vi "Value_Update_to_Preset.vi"(9 "Coordinate Array with Changes":i32[][](array[numeric]), 11 "Input Table":string[][](array[string])) -> (1 "Column Headers":string[](array[string])=["Device Name", "Device Variable", "Preset Value"], 3 "Output Table with Changes":string[][](array[string]))   [LabVIEW 2020]
uses:
  <userlib>/_OpenG.lib/array/array.llb/Empty 2D Array (I32)__ogtk.vi
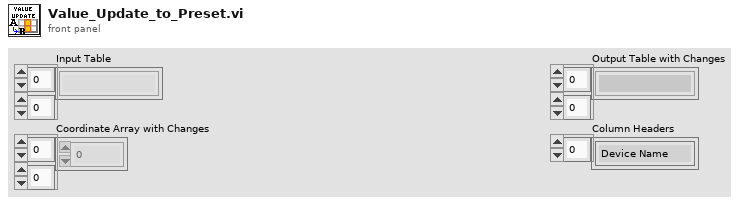
[diagram p1: front panel]
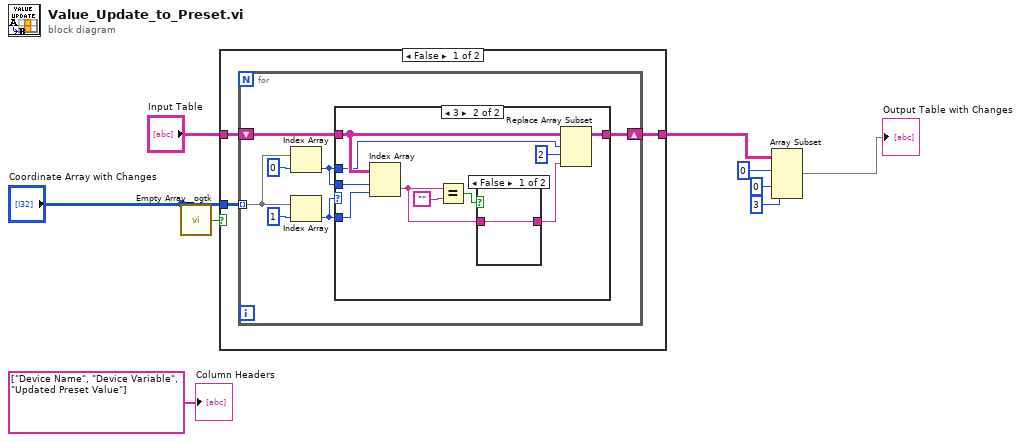
[diagram p0: block diagram]
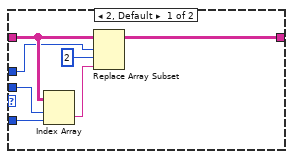
[diagram p2: hidden frame]
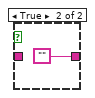
[diagram p3: hidden frame]
diagram:
  n1 = call-poly <userlib>:"Empty Array__ogtk.vi"("Array"="Coordinate Array with Changes") -> ("Empty Array?"=w9:bool)  [unwired: 8 in]
  n2 = case shown="False" w9 {
    tunnel: "Coordinate Array with Changes" -> [w12 _]
    tunnel: "Input Table" -> [w11 w39]
    tunnel: [w10 w39] -> w5
    frame False {
      n3 = for {
        tunnel: w12 -> [w19] mode=indexing
        shift-right: [w14] -> w10
        shift-left: w11 -> [w13]
        n4 = Index Array(array=w19, index=0) -> (element=w16:i32)
        n5 = Index Array(array=w19, index=1) -> (element=w15:i32)
        n6 = case shown="3" w15 {
          tunnel: w13 -> [w25 w35]
          tunnel: w16 -> [w26 w36]
          tunnel: w16 -> [w23 w34]
          tunnel: w15 -> [w21 w32]
          tunnel: [w20 w31] -> w14
          frame 2, Default {
            n7 = Index Array(array=w25, index (row)=w26, index (col)=w21) -> (element=w24:string)
            n8 = Replace Array Subset(array=w25, new element=w24, index (row)=w23, index (col)=2 ("disabled index (col)")) -> (w20:string[][])
          }
          frame 3 {
            n9 = Index Array(array=w35, index (row)=w36, index (col)=w32) -> (element=w27:string)
            n10 = Equal?(x=w27, y="") -> (x = y?=w29:bool)
            n11 = case shown="False" w29 {
              tunnel: [w37 ""] -> w28
              tunnel: w27 -> [w37 _]
              frame False {
              }
              frame True {
              }
            }
            n12 = Replace Array Subset(array=w35, new element=w28, index (row)=w34, index (col)=2 ("disabled index (col)")) -> (w31:string[][])
          }
        }
      }
    }
    frame True {
    }
  }
  n13 = Array Subset(array=w5, index (row)=0 ("index"), index (col)=0 ("index"), length (col)=3 ("length")) -> (→"Output Table with Changes":string[][])  [unwired: 1 in]
  "Column Headers" <- string[] ["Device Name", "Device Variable", "Updated Preset Value"] ("Column Headers")
